vi "GetAudioVideoFile.vi"(11 "TBSize":dbl=57336.0) -> (1 "Segments":dbl, 3 "Data":u8[](array[numeric]))   [LabVIEW 2015]
panel:
  out "size(s)":i32
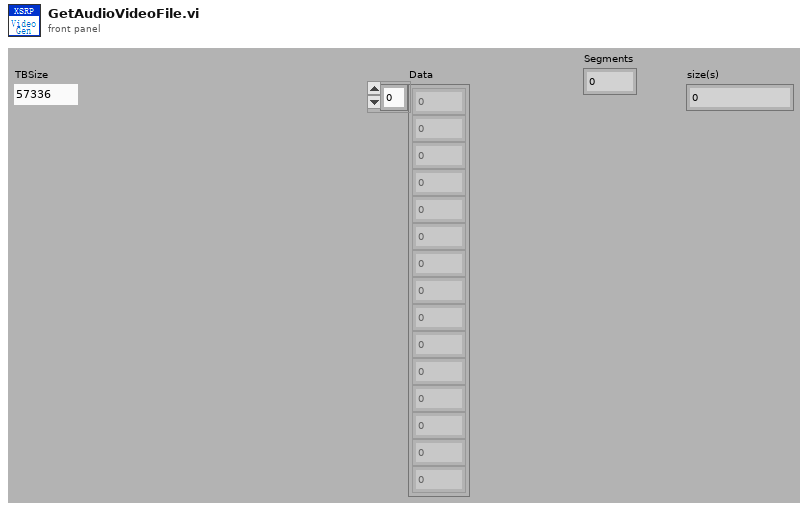
[diagram p1: front panel]
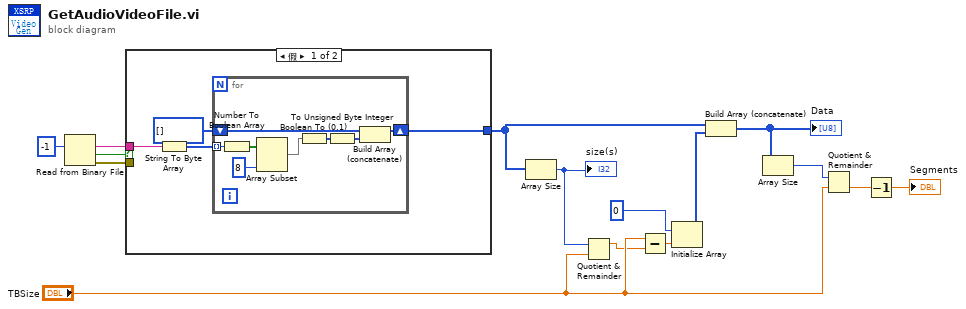
[diagram p0: block diagram]
diagram:
  n1 = Read from Binary File(10:-1 ("count (1)")) -> (0:w12:errorcluster, 1:w15:bool, 2:w14:string)  [unwired: 1 in, 5 out]
  n2 = case shown="假" w15 {
    tunnel: w14 -> [w19 _]
    tunnel: [w17 _] -> w11
    tunnel: w12 -> [_ _]
    frame False {
      n3 = String To Byte Array(string=w19) -> (unsigned byte array=w16:u8[])
      n4 = for {
        tunnel: w16 -> [w27] mode=indexing
        shift-right: [w25] -> w17
        shift-left: u8[] [] -> [w24]
        n5 = Number To Boolean Array(number=w27) -> (Boolean array=w23:bool[])
        n6 = Array Subset(array=w23, length=8) -> (w21:bool[])  [unwired: 1 in]
        n7 = Boolean To (0,1)(Boolean=w21) -> (0, 1=w26:i16[])
        n8 = To Unsigned Byte Integer(number=w26) -> (unsigned 8bit integer=w20:u8[])
        n9 = Build Array (concatenate)(w24, w20) -> (w25:u8[])
      }
    }
    frame True {
    }
  }
  n10 = Array Size(array=w11) -> (size(s)=w10:i32)
  "size(s)" <- w10
  n11 = Quotient & Remainder(x=w10, y="TBSize") -> (x-y*floor(x/y)=w1:dbl)  [unwired: 1 out]
  n12 = Subtract(x="TBSize", y=w1) -> (x-y=w2:dbl)
  n13 = Initialize Array(u8 0 ("element"), w2) -> (w8:u8[])
  n14 = Build Array (concatenate)(w11, w8) -> (w7:u8[])
  "Data" <- w7
  n15 = Array Size(array=w7) -> (size(s)=w6:i32)
  n16 = Quotient & Remainder(x=w6, y="TBSize") -> (floor(x/y)=w5:dbl)  [unwired: 1 out]
  n17 = Decrement(x=w5) -> (x-1=→"Segments":dbl)
